vi "Find_Variable.vi"(2 "Input string":string, 3 "Variable name":string) -> (0 "No Match?":bool, 1 "After  Matched string":string)   [LabVIEW 2021]
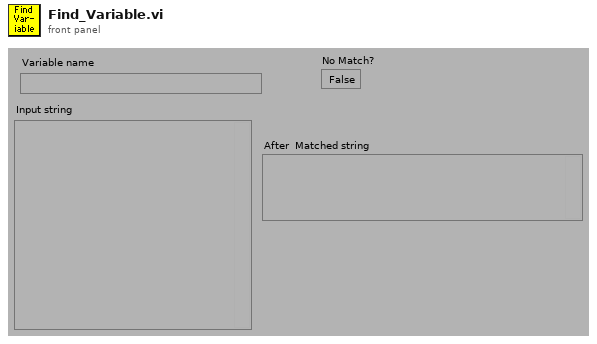
[diagram p1: front panel]
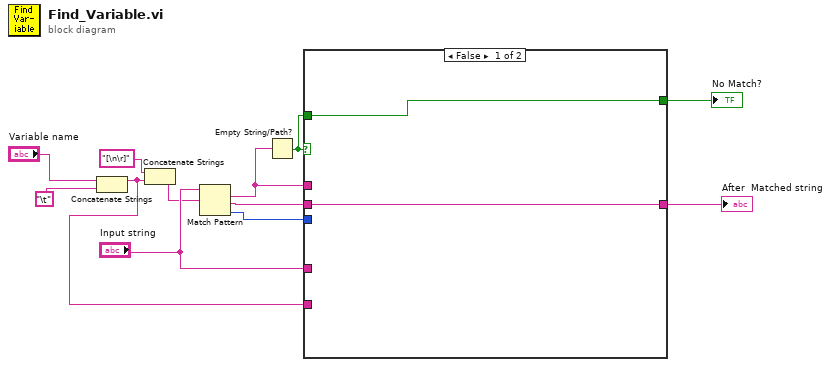
[diagram p0: block diagram]
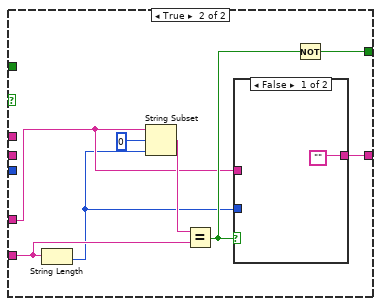
[diagram p2: hidden frame]
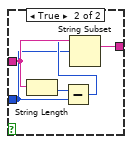
[diagram p3: hidden frame]
diagram:
  n1 = Concatenate Strings("Variable name", "\t") -> (w1:string)
  n2 = Concatenate Strings("[\n\r]" ("x"), w1) -> (w2:string)
  n3 = Match Pattern(string="Input string", regular expression=w2) -> (match substring=w7:string, after substring=w10:string, offset past match=w8:i32)  [unwired: 2 out]
  n4 = Empty String/Path?(string/path=w7) -> (empty?=w6:bool)
  n5 = case shown="False" w6 {
    tunnel: w10 -> [w14 _]
    tunnel: [w14 w17] -> w9
    tunnel: w7 -> [_ _]
    tunnel: w8 -> [_ _]
    tunnel: w6 -> [w13 _]
    tunnel: [w13 w18] -> w5
    tunnel: "Input string" -> [_ w16]
    tunnel: w1 -> [_ w22]
    frame False {
    }
    frame True {
      n6 = String Length(string=w22) -> (length=w15:i32)
      n7 = String Subset(string=w16, offset (0)=0, length (rest)=w15) -> (substring=w20:string)
      n8 = Equal?(x=w20, y=w22) -> (x = y?=w19:bool)
      n9 = case shown="False" w19 {
        tunnel: ["" w24] -> w17
        tunnel: w16 -> [_ w28]
        tunnel: w15 -> [_ w25]
        frame False {
        }
        frame True {
          n10 = String Length(string=w28) -> (length=w27:i32)
          n11 = Subtract(x=w27, y=w25) -> (x-y=w26:i32)
          n12 = String Subset(string=w28, offset (0)=w25, length (rest)=w26) -> (substring=w24:string)
        }
      }
      n13 = Not(x=w19) -> (.not. x?=w18:bool)
    }
  }
  "No Match?" <- w5
  "After  Matched string" <- w9
